vi "ATM_TakeAction.vi"(4 "User Input":dbl, 5 "Balance":dbl, 6 "Action Type":string) -> (0 "ATM Message":string, 1 "New Balance":dbl, 2 "Enum":T1=enum."Idle")   [LabVIEW 2020]
uses:
  Enum (Client).ctl
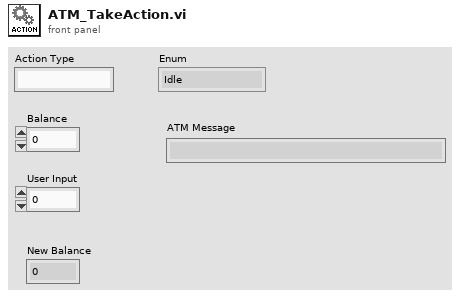
[diagram p1: front panel]
types:
  T1 = typedef "Enum (Client).ctl" = enum16{"Start", "Idle", "Actions", "Empty Check", "Data Transmission", "Update File"}
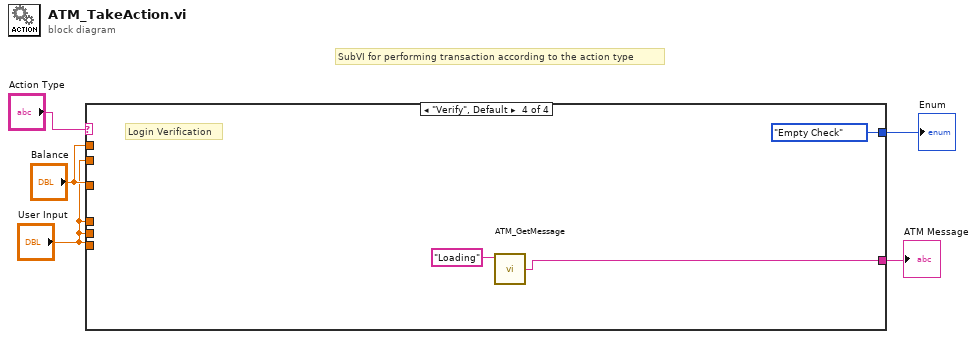
[diagram p0: block diagram]
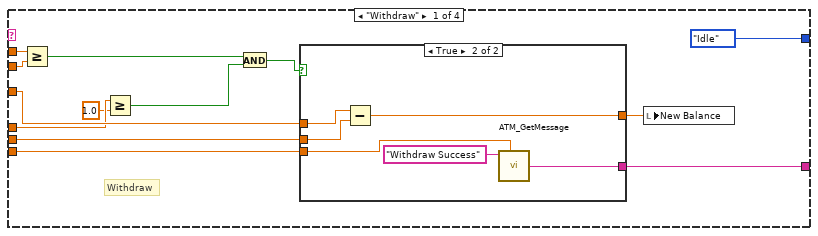
[diagram p2: hidden frame]
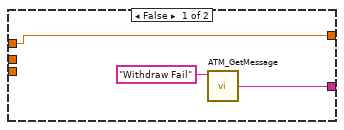
[diagram p3: hidden frame]
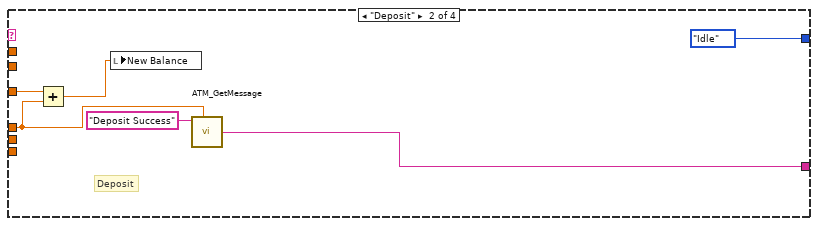
[diagram p4: hidden frame]
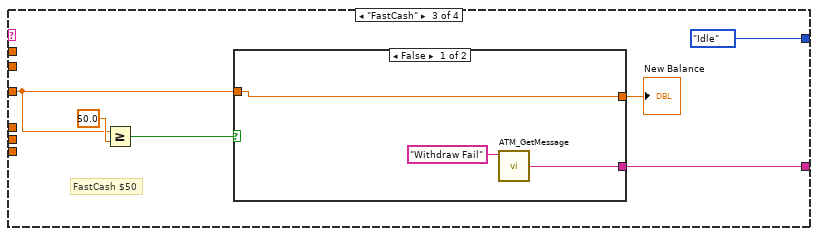
[diagram p5: hidden frame]
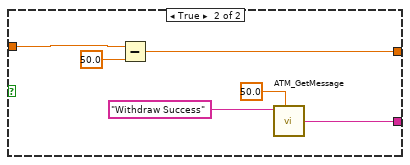
[diagram p6: hidden frame]
diagram:
  # "SubVI for performing transaction according to the action type"
  n1 = case shown="\"Verify\", Default" "Action Type" {
    tunnel: [Enum_(Client)."Idle" Enum_(Client)."Idle" Enum_(Client)."Idle" Enum_(Client)."Empty Check"] -> w4
    tunnel: "Balance" -> [w18 _ _ _]
    tunnel: "User Input" -> [w17 _ _ _]
    tunnel: "Balance" -> [w16 w32 w35 _]
    tunnel: "User Input" -> [w15 _ _ _]
    tunnel: "User Input" -> [w12 w30 _ _]
    tunnel: "User Input" -> [w7 _ _ _]
    tunnel: [w6 w28 w34 w49] -> w1
    frame "Withdraw" {
      # "Withdraw"
      n2 = Greater Or Equal?(x=w18, y=w17) -> (x >= y?=w9:bool)
      n3 = Greater Or Equal?(x=w12, y=1.0) -> (x >= y?=w8:bool)
      n4 = And(x=w9, y=w8) -> (x .and. y?=w10:bool)
      n5 = case shown="True" w10 {
        tunnel: w16 -> [w19 w27]
        tunnel: w15 -> [_ w26]
        tunnel: w7 -> [_ w25]
        tunnel: [w20 w23] -> w6
        tunnel: [w19 w22] -> w13
        frame False {
          n6 = call "ATM_GetMessage.vi"("Message Type"="Withdraw Fail") -> ("ATM Message"=w20:string)  [unwired: 4 in]
        }
        frame True {
          n7 = Subtract(x=w27, y=w26) -> (x-y=w22:dbl)
          n8 = call "ATM_GetMessage.vi"("Message Type"="Withdraw Success", "User Input"=w25) -> ("ATM Message"=w23:string)  [unwired: 3 in]
        }
      }
      n9 = local write "New Balance"(w13) -> ()
    }
    frame "Deposit" {
      # "Deposit"
      n10 = Add(x=w32, y=w30) -> (x+y=w29:dbl)
      n11 = local write "New Balance"(w29) -> ()
      n12 = call "ATM_GetMessage.vi"("Message Type"="Deposit Success", "User Input"=w30) -> ("ATM Message"=w28:string)  [unwired: 3 in]
    }
    frame "FastCash" {
      # "FastCash $50"
      n13 = Greater Or Equal?(x=w35, y=50.0) -> (x >= y?=w37:bool)
      n14 = case shown="False" w37 {
        tunnel: w35 -> [w40 w44]
        tunnel: [w41 w47] -> w34
        tunnel: [w40 w46] -> w36
        frame False {
          n15 = call "ATM_GetMessage.vi"("Message Type"="Withdraw Fail") -> ("ATM Message"=w41:string)  [unwired: 4 in]
        }
        frame True {
          n16 = Subtract(x=w44, y=50.0) -> (x-y=w46:dbl)
          n17 = call "ATM_GetMessage.vi"("Message Type"="Withdraw Success", "User Input"=50.0) -> ("ATM Message"=w47:string)  [unwired: 3 in]
        }
      }
      "New Balance" <- w36
    }
    frame "Verify", Default {
      # "Login Verification"
      n18 = call "ATM_GetMessage.vi"("Message Type"="Loading") -> ("ATM Message"=w49:string)  [unwired: 4 in]
    }
  }
  "Enum" <- w4
  "ATM Message" <- w1
